vi "DBM Reg Req.vi"(8 "에러 입력(에러 없음)":errorcluster) -> (0 "에러 출력":errorcluster, 2 "모델 요청 갯수":u8, 3 "기준기 요청 갯수":u8, 4 "모델요청":string[][](array[string]), 5 "기준기요청":string[][](array[string]))   [LabVIEW 2020]
uses:
  Controls/Cmd_Read Query.ctl
  Controls/Clst_Query Info.ctl
  <vilib>/addons/database/NI_Database_API.lvlib
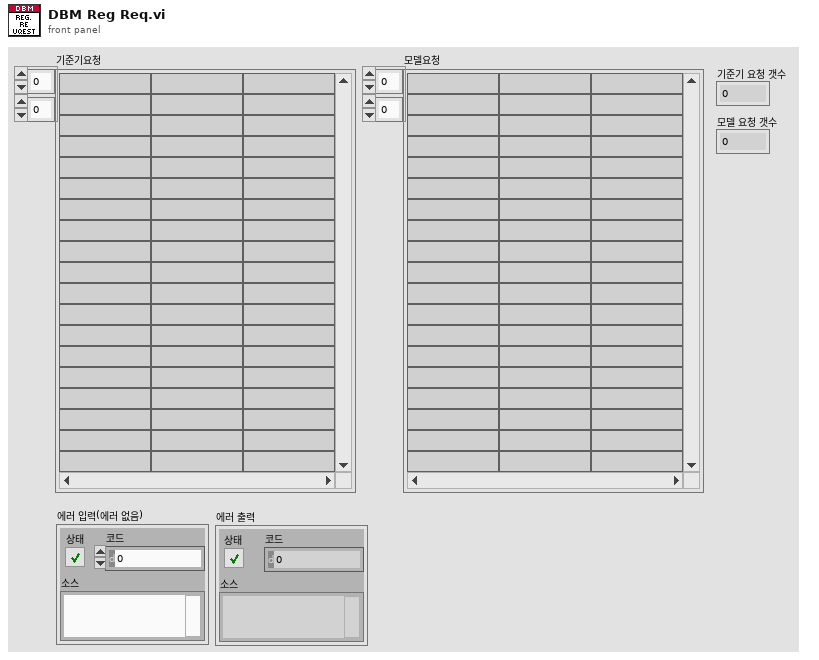
[diagram p1: front panel]
types:
  T1 = typedef "Cmd_Read Query.ctl" = enum16{"교정자 이름 얻기", "인증교정자 얻기", "기술책임자 얻기", "기책부책 얻기", "등록번호 얻기", "등록정보 얻기", "업체정보 얻기", "교정일자(CAMAS) 얻기", "교정일자(CALSTD) 얻기", "교정환경 얻기", "교정절차서 목록 얻기", "교정절차서명 얻기", "교정절차 목록얻기", "교정절차 얻기", "PROC 교정절차 얻기", "PROC SPEC 얻기", "교정절차(Func별) 얻기", "교정절차(Func_ext별) 얻기", "기관코드 얻기", "교정기능(세부분류) 얻기", "교정기능(모델) 얻기", "교정기능 목록 얻기", "교정기능 명칭 얻기", "교정기능 항목명칭 얻기", "DB (사용기준기) 얻기", "DB (기준기이름) 얻기", "DB (기준기이름목록) 얻기", "DB (기준기목록) 얻기", "DB (기준기값) 얻기", "DB (CMC) 얻기", "DB (FUNC) 얻기", "DB (CALNAME) 얻기", "DB (STDNAME) 얻기", "DB (SPEC) 얻기", "모델(항목전체) 얻기", "모델(최대범위) 얻기", "모델(최소범위) 얻기", "모델(최대최소) 얻기", "모델(범위조건) 얻기", "모델(등록요청) 얻기", "모델(형식별) 얻기", "모델(조건별) 얻기", "모델(모델검색) 얻기", "세부분류 목록 얻기", "기준기등록리스트 얻기", "STD Cal Date Check", "DB등록일자 얻기", "적용항목 얻기", "기타정보 얻기", "기준기요청 얻기", "서버버전 얻기"}
  T2 = typedef "Clst_Query Info.ctl" = cluster{"사번":string, "등록번호":string, "업체명":string, "세부분류코드":string, "형식":string, "기기번호":string, "FUNC":string, "FUNC_EXT":string, "옵션":string, "추가문자열":string, "일자":string, "배열 1":string[], "배열 2":string[], "항목명":string, "문자열":string, "이름":string}
  T3 = typedef "NI_Database_API.lvlib/Conn ObjectReference.ctl" = refnum<k1>
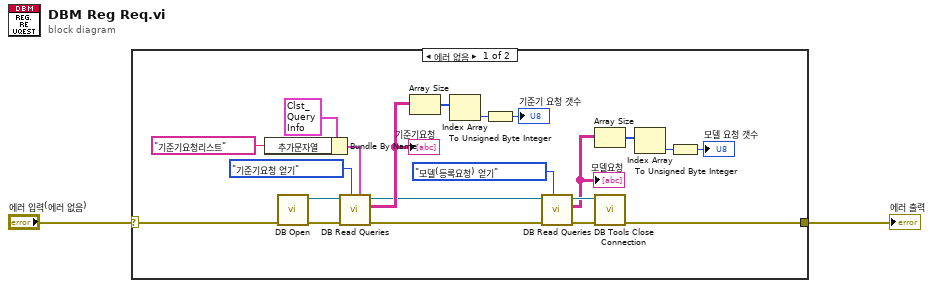
[diagram p0: block diagram]
diagram:
  n1 = case shown="에러 없음" "에러 입력(에러 없음)" {
    selector: "에러 입력(에러 없음)" -> [w17 w24]
    tunnel: [w16 w24] -> w1
    frame No Error {
      n2 = Bundle By Name(cluster=T2 {"사번"="", "등록번호"="", "업체명"="", "세부분류코드"="", "형식"="", "기기번호"="", "FUNC"="", "FUNC_EXT"="", "옵션"="", "추가문자열"="", "일자"="", "배열 1"=[], "배열 2"=[], "항목명"="", "문자열"="", "이름"=""} ("Query info"), "추가문자열"="기준기요청리스트") -> (w22:T2)
      n3 = call "DB Open.vi"("에러 입력"=w17) -> ("에러 출력"=w18:errorcluster, "참조 번호 출력"=w19:T3)  [unwired: 9 in]
      n4 = call "DB Read Queries.vi"("Query info"=w22, "Query Command"=Cmd_Read_Query."기준기요청 얻기", "에러 입력(에러 없음)"=w18, "참조 번호 입력"=w19) -> ("에러 출력"=w10:errorcluster, "Data"=w15:string[][], "참조 번호 출력"=w9:T3)  [unwired: 3 in, 2 out]
      "기준기요청" <- w15
      n5 = Array Size(array=w15) -> (size(s)=w14:i32[])
      n6 = Index Array(array=w14) -> (element=w13:i32)  [unwired: 1 in]
      n7 = To Unsigned Byte Integer(number=w13) -> (unsigned 8bit integer=→"기준기 요청 갯수":u8)
      n8 = call "DB Read Queries.vi"("Query Command"=Cmd_Read_Query."모델(등록요청) 얻기", "에러 입력(에러 없음)"=w10, "참조 번호 입력"=w9) -> ("에러 출력"=w7:errorcluster, "Data"=w3:string[][], "참조 번호 출력"=w8:T3)  [unwired: 4 in, 2 out]
      "모델요청" <- w3
      n9 = Array Size(array=w3) -> (size(s)=w4:i32[])
      n10 = call <vilib>:"DB Tools Close Connection.vi"("error in (no error)"=w7, "connection reference"=w8) -> ("error out"=w16:errorcluster)  [unwired: 5 in]
      n11 = Index Array(array=w4) -> (element=w5:i32)  [unwired: 1 in]
      n12 = To Unsigned Byte Integer(number=w5) -> (unsigned 8bit integer=→"모델 요청 갯수":u8)
    }
    frame Error {
    }
  }
  "에러 출력" <- w1
